vi "FFT Test.vi"   [LabVIEW 2014]
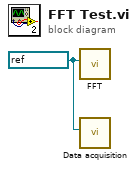
[diagram p0: block diagram]
diagram:
  w1 = refnum<k21> "50MHz" ("Timing Source")
  n1 = call "FFT.vi"("Timing Source"=w1) -> ()  [unwired: 11 in]
  n2 = call "Data acquisition.vi"("Timing Source"=w1) -> ()  [unwired: 10 in, 1 out]
